vi "Injection Capture Core.vi"(7 "FIFOs":T2={"Data FIFO"="Intermediate Voltage 0", "Trigger FIFO"="Event Capture 0"}, 8 "Current (PreScaled)":fxp<+/-,32,8>, 9 "Voltage (PreScaled)":fxp<+/-,32,8>, 10 "Settings.Index<#>.<UserName>":T1, 11 "Settings.Global":T3={"Enable?"=FALSE, "Initial Voltage Threshold"=12.0, "Event Dwell Limit"=2000, "Voltage Gain"=1.0, "Current Gain"=1.0}) -> (0 "Current (Scaled)":fxp<+/-,32,8>, 1 "Voltage (Scaled)":fxp<+/-,32,8>, 3 "Intermediate FIFO Timeout?":bool)   [LabVIEW 2015]
uses:
  Types/Injection.Global.Settings.ctl
  Types/Injection.Core.Internal.Settings.ctl
  Types/Injection.Core.Settings.ctl
  <vilib>/rvi/DataTransferAndStorage/Container/Common/niFpgaContainerExecOnDevCompGetState.vi
  <vilib>/rvi/Emulation/niFpgaEmulationIsFPGAContextNoSignature.vi
  <vilib>/rvi/Emulation/niFpgaSctlEmulationGetInTimedLoop.vi
  <vilib>/rvi/errors/niFpgaSetErrorForExecOnDevCompSimple.vi
  <vilib>/rvi/eio/common/nirviEmuReportErrorAndStop.vi
  <vilib>/rvi/DataTransferAndStorage/Container/Common/niFpgaContainerGetUniqueNameForEmu.vi
  <vilib>/rvi/FIFO/Fifo_Resource/nirvififoEmulationSetSize.vi
  <vilib>/rvi/FIFO/Fifo_Resource/nirviFifoEmulationQueueMgr.vi
  <instcachedir>/0/nirviFifoEmulationQueueMgr_E5CAEC123FF24DC58D834DCA3CDAA9B5.lvgen/nirviFifoEmulationQueueMgr_E5CAEC123FF24DC58D834DCA3CDAA9B5_010.vi
  <vilib>/rvi/FIFO/Fifo_Resource/nirvififoEmulationDetermineInputValidOut.vi
  <vilib>/rvi/FIFO/Fifo_Resource/nirvififoEmulationCreateLock.vi
  <vilib>/rvi/Emulation/niFpgaProcessEmulError.vi
  <vilib>/rvi/FIFO/Fifo_Resource/nirvififoEmulationObtainLock.vi
  <vilib>/rvi/FIFO/Fifo_Resource/nirvififoEmulationReleaseLock.vi
  <vilib>/rvi/occurrence/nirviWaitOnOccurrenceBase.vi
  <vilib>/rvi/errors/nirviReportUnexpectedCaseInternalError.vi
  <vilib>/rvi/errors/nirviReportUnexpectedCaseInternalError (U32).vi
  <vilib>/Utility/error.llb/Clear Errors.vi
  <vilib>/rvi/interface/RandomDataEmulation/niFpgaRandomDataHandleErrors.vi
  <instcachedir>/0/nirviFifoEmulationQueueMgr_E5CAEC123FF24DC58D834DCA3CDAA9B5.lvgen/nirviFifoEmulationQueueMgr_E5CAEC123FF24DC58D834DCA3CDAA9B5_008.vi
  <vilib>/rvi/DataTransferAndStorage/Container/XNode/niFpgaContainer.xnode
  <vilib>/rvi/FIFO/Fifo_Resource/niFpgaFifoEmulationRefIn.vi
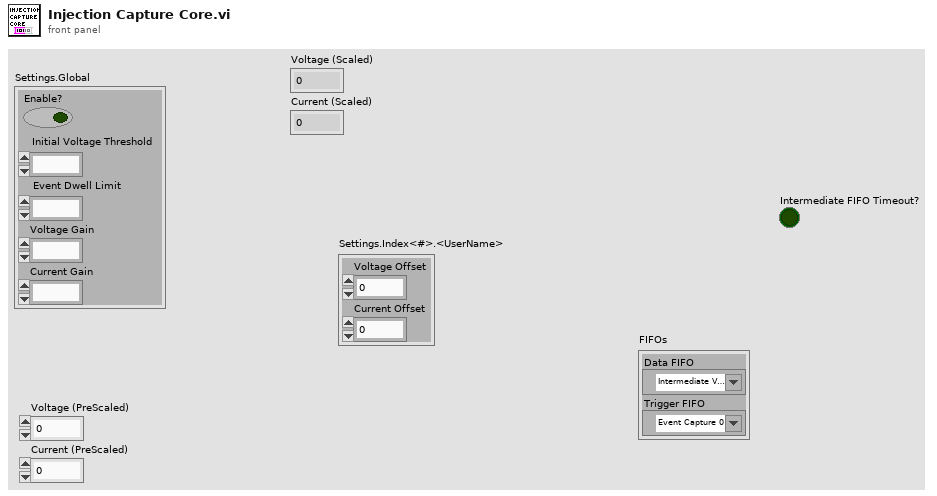
[diagram p1: front panel]
types:
  T1 = typedef "Injection.Core.Settings.ctl" = cluster{"Voltage Offset":fxp<+/-,32,8>, "Current Offset":fxp<+/-,32,8>}
  T2 = typedef "Injection.Core.Internal.Settings.ctl" = cluster{"Data FIFO":refnum<k21>, "Trigger FIFO":refnum<k21>}
  T3 = typedef "Injection.Global.Settings.ctl" = cluster{"Enable?":bool, "Initial Voltage Threshold":fxp<+/-,32,8>, "Event Dwell Limit":u16, "Voltage Gain":fxp<+/-,32,8>, "Current Gain":fxp<+/-,32,8>}
  T4 = cluster{"Event.Count":u16, "Injection.Period":u32, "Injection.CachedPeriod":u32}
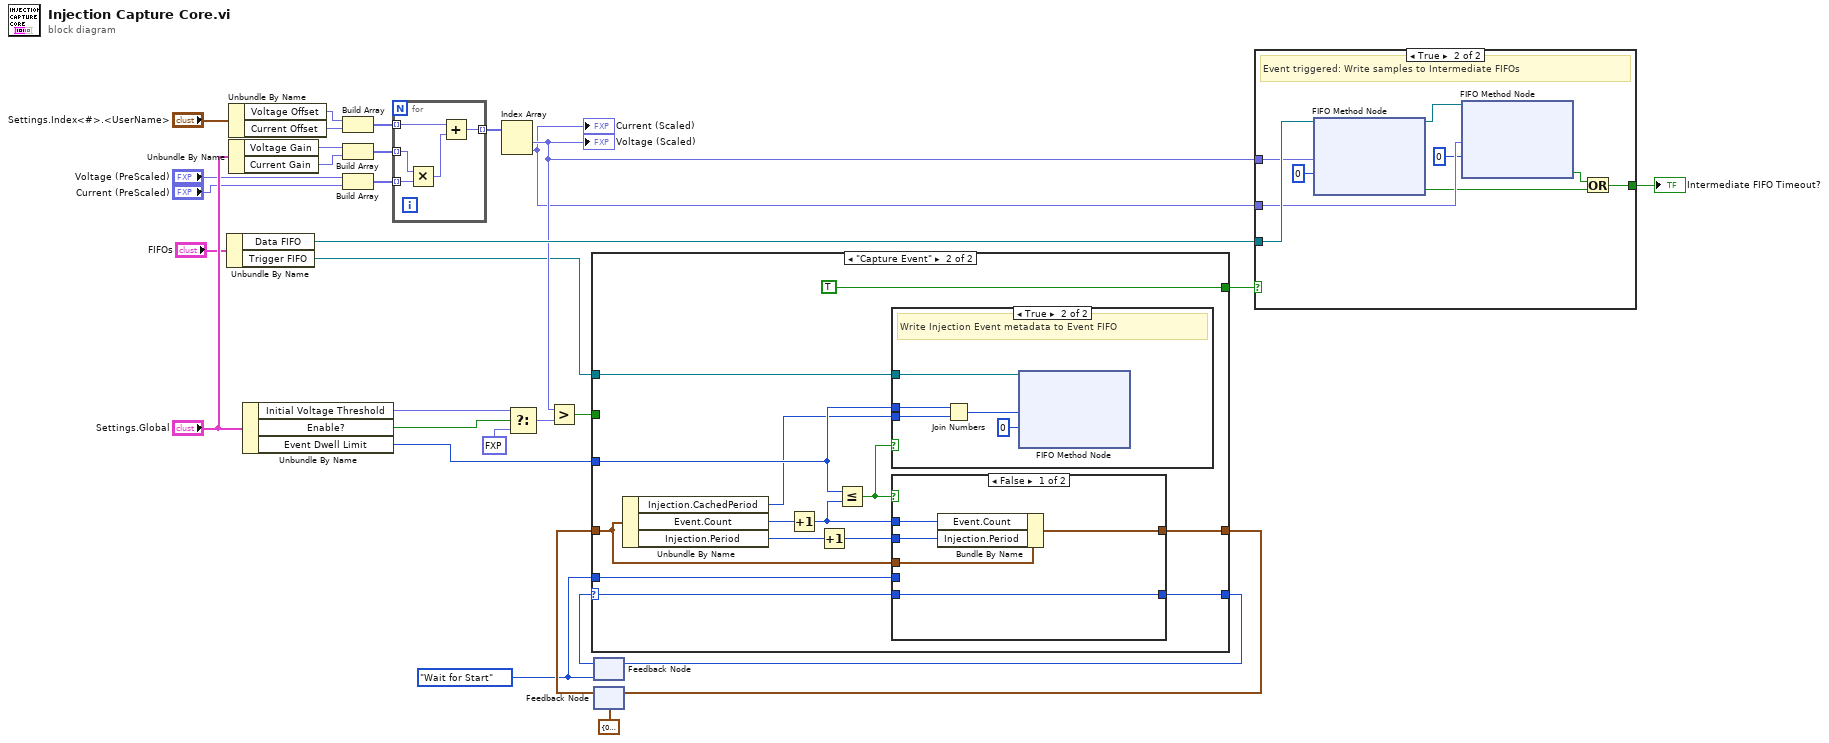
[diagram p0: block diagram]
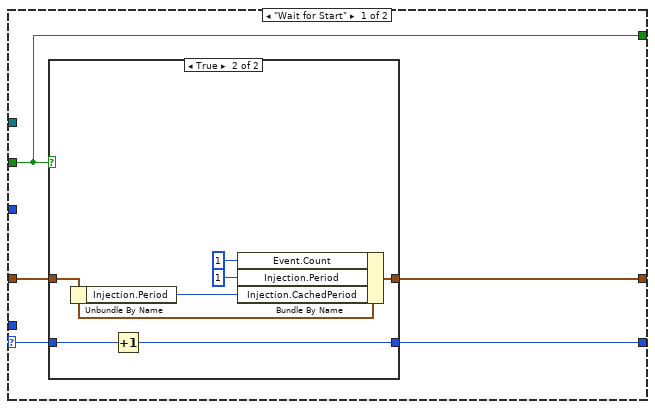
[diagram p2: hidden frame]
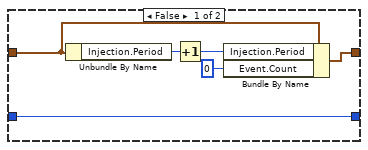
[diagram p3: hidden frame]
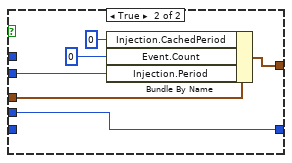
[diagram p5: hidden frame]
diagram:
  w14 = enum8{"Wait for Start", "Capture Event"}."Wait for Start"
  n1 = Unbundle By Name("FIFOs") -> ("Data FIFO"=w27:refnum<k21>, "Trigger FIFO"=w1:refnum<k21>)
  n2 = Unbundle By Name("Settings.Index<#>.<UserName>") -> ("Voltage Offset"=w10:fxp<+/-,32,8>, "Current Offset"=w11:fxp<+/-,32,8>)
  n3 = Unbundle By Name("Settings.Global") -> ("Voltage Gain"=w12:fxp<+/-,32,8>, "Current Gain"=w8:fxp<+/-,32,8>)
  n4 = Unbundle By Name("Settings.Global") -> ("Initial Voltage Threshold"=w23:fxp<+/-,32,8>, "Enable?"=w25:bool, "Event Dwell Limit"=w17:u16)
  n5 = Build Array(w10, w11) -> (w9:fxp<+/-,32,8>[])
  n6 = Build Array(w12, w8) -> (w7:fxp<+/-,32,8>[])
  n7 = Build Array("Voltage (PreScaled)", "Current (PreScaled)") -> (w5:fxp<+/-,32,8>[])
  n8 = for {
    tunnel: w5 -> [w36] mode=indexing
    tunnel: [w35] -> w4 mode=indexing
    tunnel: w9 -> [w33] mode=indexing
    tunnel: w7 -> [w32] mode=indexing
    n9 = Multiply(x=w32, y=w36) -> (x*y=w34:fxp<+/-,32,8>)
    n10 = Add(x=w33, y=w34) -> (x+y=w35:fxp<+/-,32,8>)
  }
  n11 = Index Array(array=w4) -> (element #1=w3:fxp<+/-,32,8>, element #2=w2:fxp<+/-,32,8>)  [unwired: 2 in]
  "Current (Scaled)" <- w2
  "Voltage (Scaled)" <- w3
  n12 = Select(t=w23, s=w25, f=fxp<+/-,32,8> 127.99999994039536) -> (s? t:f=w26:fxp<+/-,32,8>)
  n13 = Greater?(x=w3, y=w26) -> (0:w21:bool)
  n14 = feedback #1(w14) -> (w22:enum8{"Wait for Start", "Capture Event"})
  n15 = feedback #2(T4 {"Event.Count"=0, "Injection.Period"=0, "Injection.CachedPeriod"=0}) -> (w19:T4)
  n16 = case shown="\"Capture Event\"" w22 {
    selector: w22 -> [w40 w60]
    tunnel: w21 -> [w38 _]
    tunnel: w19 -> [w41 w66]
    tunnel: [w39 w62] -> w18
    tunnel: w17 -> [_ w57]
    tunnel: [w38 TRUE] -> w16
    tunnel: [w37 w64] -> w15
    tunnel: w14 -> [_ w61]
    tunnel: w1 -> [_ w59]
    frame "Wait for Start" {
      n17 = case shown="True" w38 {
        tunnel: w41 -> [w46 w52]
        tunnel: w40 -> [w47 w54]
        tunnel: [w47 w53] -> w39
        tunnel: [w45 w50] -> w37
        frame False {
          n18 = Unbundle By Name(w46) -> ("Injection.Period"=w43:u32)
          n19 = Increment(x=w43) -> (x+1=w44:u32)
          n20 = Bundle By Name(cluster=w46, "Injection.Period"=w44, "Event.Count"=u32 0) -> (w45:T4)
        }
        frame True {
          n21 = Unbundle By Name(w52) -> ("Injection.Period"=w48:u32)
          n22 = Increment(x=w54) -> (x+1=w53:enum8{"Wait for Start", "Capture Event"})
          n23 = Bundle By Name(cluster=w52, "Event.Count"=u16 1, "Injection.Period"=u32 1 ("Event.Count"), "Injection.CachedPeriod"=w48) -> (w50:T4)
        }
      }
    }
    frame "Capture Event" {
      n24 = Unbundle By Name(w66) -> ("Injection.CachedPeriod"=w55:u32, "Event.Count"=w68:u16, "Injection.Period"=w67:u32)
      n25 = Increment(x=w68) -> (x+1=w63:u16)
      n26 = Increment(x=w67) -> (x+1=w65:u32)
      n27 = Less Or Equal?(x=w57, y=w63) -> (x <= y?=w58:bool)
      n28 = case shown="True" w58 {
        tunnel: w57 -> [_ w70]
        tunnel: w59 -> [_ w73]
        tunnel: w55 -> [_ w71]
        frame False {
        }
        frame True {
          # "Write Injection Event metadata to Event FIFO"
          n29 = Join Numbers(hi=w70, lo=w71) -> ((hi.lo)=w69:u64)
          n30 = xnode ("FIFO Method Node")("Element"=w69, "Timeout"=0, "FIFO In"=w73) -> ()  [unwired: 2 out]
        }
      }
      n31 = case shown="False" w58 {
        tunnel: w66 -> [w78 w84]
        tunnel: w65 -> [w77 w82]
        tunnel: [w76 w83] -> w64
        tunnel: w63 -> [w75 _]
        tunnel: [w74 w80] -> w62
        tunnel: w61 -> [_ w80]
        tunnel: w60 -> [w74 _]
        frame False {
          n32 = Bundle By Name(cluster=w78, "Event.Count"=w75, "Injection.Period"=w77) -> (w76:T4)
        }
        frame True {
          n33 = Bundle By Name(cluster=w84, "Injection.CachedPeriod"=u32 0, "Event.Count"=u16 0, "Injection.Period"=w82) -> (w83:T4)
        }
      }
    }
  }
  n34 = feedback-in #1(w18) -> ()
  n35 = feedback-in #2(w15) -> ()
  n36 = case shown="True" w16 {
    tunnel: w3 -> [_ w86]
    tunnel: [_ w88] -> w29
    tunnel: w2 -> [_ w91]
    tunnel: w27 -> [_ w92]
    frame False {
      # "Event is not triggered"
    }
    frame True {
      # "Event triggered: Write samples to Intermediate FIFOs"
      n37 = xnode ("FIFO Method Node")("Element"=w86, "Timeout"=0 ("timeout in ms (0)"), "FIFO In"=w92) -> ("Timed Out?"=w89:bool, "FIFO Out"=w85:refnum<k21>)  [unwired: 1 in, 1 out]
      n38 = xnode ("FIFO Method Node")("Element"=w91, "Timeout"=0 ("timeout in ms (0)"), "FIFO In"=w85) -> ("Timed Out?"=w87:bool)  [unwired: 1 in, 2 out]
      n39 = Or(x=w87, y=w89) -> (x .or. y?=w88:bool)
    }
  }
  "Intermediate FIFO Timeout?" <- w29
